vi "read.vi"(8 "error in (no error)":errorcluster, 10 "ElectrometerController in":refnum<class "ElectrometerController.lvclass">, 11 "SetDurationReading in":refnum<class "SetDurationReading.lvclass">) -> (0 "error out":errorcluster, 1 "lastMeasure":dbl, 2 "ElectrometerController out":refnum<class "ElectrometerController.lvclass">, 3 "SetDurationReading out":refnum<class "SetDurationReading.lvclass">)   [LabVIEW 2016, in "SetDurationReading.lvclass"]
uses:
  SetDurationReading.lvclass
  ElectrometerController/ElectrometerController.lvclass
  State.lvclass
  Electrometer.lvclass
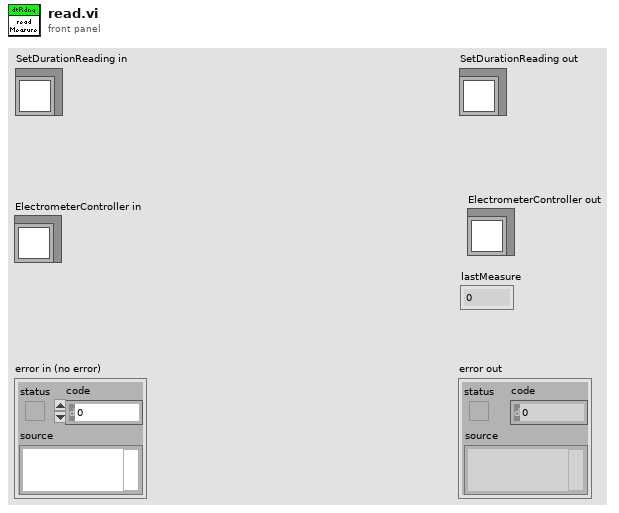
[diagram p1: front panel]
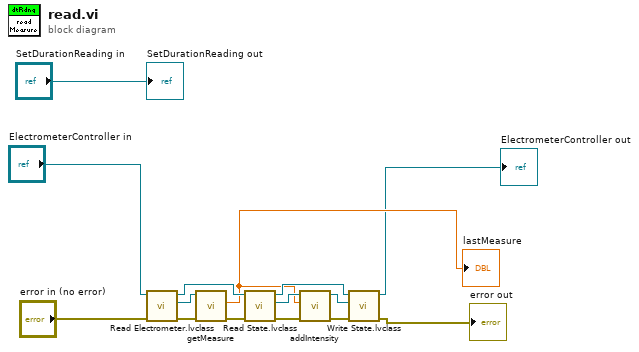
[diagram p0: block diagram]
diagram:
  n1 = call-dynamic "Read Electrometer.lvclass.vi"("error in (no error)"="error in (no error)", "ElectrometerController in"="ElectrometerController in") -> ("error out"=w13:errorcluster, "Electrometer.lvclass"=w14:refnum<class "Electrometer.lvclass">, "ElectrometerController out"=w12:refnum<class "ElectrometerController.lvclass">)  [unwired: 7 in]
  n2 = call "getMeasure.vi"("error in (no error)"=w13, "Electrometer in"=w14) -> ("error out"=w11:errorcluster, "Measure"=w5:dbl)  [unwired: 7 in, 1 out]
  "lastMeasure" <- w5
  n3 = call-dynamic "Read State.lvclass.vi"("error in (no error)"=w11, "ElectrometerController in"=w12) -> ("error out"=w10:errorcluster, "State.lvclass"=w9:refnum<class "State.lvclass">, "ElectrometerController out"=w6:refnum<class "ElectrometerController.lvclass">)  [unwired: 7 in]
  n4 = call-dynamic "addIntensity.vi"("error in (no error)"=w10, "lastMeasure"=w5, "State in"=w9) -> ("error out"=w8:errorcluster, "State out"=w7:refnum<class "State.lvclass">)  [unwired: 7 in]
  n5 = call-dynamic "Write State.lvclass.vi"("error in (no error)"=w8, "State.lvclass"=w7, "ElectrometerController in"=w6) -> ("error out"=→"error out":errorcluster, "ElectrometerController out"=→"ElectrometerController out":refnum<class "ElectrometerController.lvclass">)  [unwired: 7 in]
  "SetDurationReading out" <- "SetDurationReading in"
